vi "placeholder--alias.vi"() -> (2 "Prefix":string)   [LabVIEW 2025, in "TEMPLATE Actor.lvlib" / "TEMPLATE Actor.lvclass"]
uses:
  TEMPLATE Actor.lvclass
  <vilib>/Nathan Davis/jettl/jettl/jettl/Actor/--X.ctl
  <vilib>/Nathan Davis/jettl/jettl/jettl/Actor/Actor.lvlib
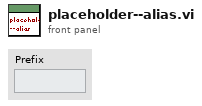
[diagram p1: front panel]
types:
  T1 = typedef "jettl.lvlib/Actor.lvlib/--X.ctl" = enum16{"--alias", "--create", "--error"}
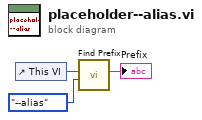
[diagram p0: block diagram]
diagram:
  n1 = control-ref of="This VI"() -> (w3:refnum<vi>)
  n2 = call <vilib>:"Find Prefix.vi"("--X"=--X."--alias", "VI Ref"=w3) -> ("Prefix"=→"Prefix":string)  [unwired: 9 in]
